vi "Read Tests.vi"() -> ()   [LabVIEW 2020]
uses:
  <vilib>/ActorFramework/Actor/Actor.lvclass
  FGV Map/Get Data/FGV Map Get Data (Variant).vi
  FGV Map/Get Data/FGV Map Get Data (String).vi
  FGV Map/Get Data/FGV Map Get Data (Bool).vi
  FGV Map/Get Data/FGV Map Get Data (DBL).vi
  FGV Map/Get Data/FGV Map Get Data (U32).vi
  FGV Map/Get Data/FGV Map Get Data (I32).vi
  FGV Map/Get Data/FGV Map Get Data (Path).vi
  FGV Map/Get Data/FGV Map Get Data (Class).vi
  FGV Map.lvlib
panel:
  out "Class2":bool
  out "Class1":bool
  out "Path":bool
  out "I32":bool
  out "U32":bool
  out "DBL":bool
  out "Bool":bool
  out "String":bool
  out "Variant":bool
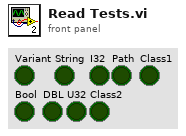
[diagram p1: front panel]
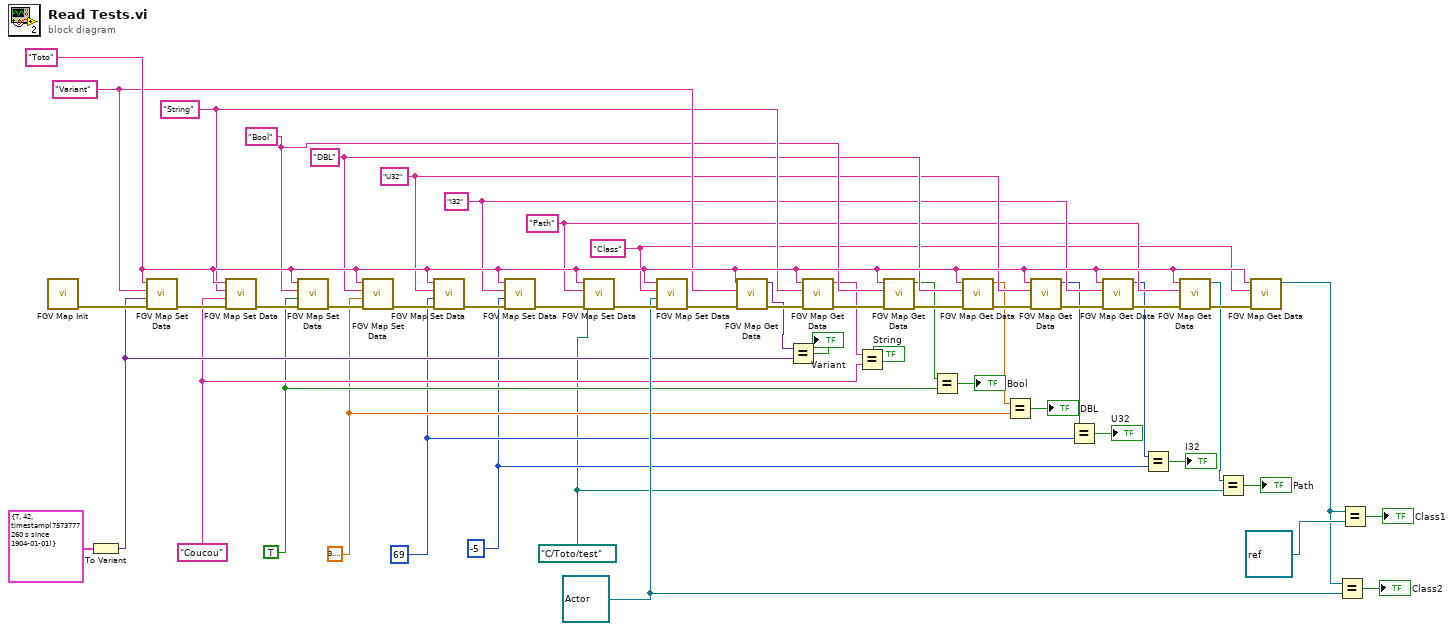
[diagram p0: block diagram]
diagram:
  w24 = refnum<class "Actor.lvclass"> refnum ("Actor")
  w27 = "Class" ("Data Key")
  w10 = path "C:/Toto/test"
  w14 = u32 69
  w12 = -5
  w16 = 3.141592653589793
  w18 = TRUE
  w20 = "Coucou"
  w28 = "Path" ("Data Key")
  w29 = "I32" ("Data Key")
  w30 = "U32" ("Data Key")
  w31 = "DBL" ("Instance Key")
  w32 = "Bool" ("Data Key")
  w33 = "String" ("Data Key")
  w34 = "Variant" ("Data Key")
  w35 = "Toto" ("Instance Key")
  n1 = call "FGV Map Init.vi"() -> ("error out"=w52:errorcluster)  [unwired: 11 in]
  n2 = To Variant(anything=cluster{bool, i32, timestamp} {TRUE, 42, timestamp(7573777260 s since 1904-01-01)}) -> (Variant=w22:variant)
  n3 = call "FGV Map Set Data.vi"("error in (no error)"=w52, "Data In"=w22, "Data Key"=w34, "Instance Key"=w35) -> ("error out"=w51:errorcluster)  [unwired: 5 in, 2 out]
  n4 = call "FGV Map Set Data.vi"("error in (no error)"=w51, "Data In"=w20, "Data Key"=w33, "Instance Key"=w35) -> ("error out"=w50:errorcluster)  [unwired: 5 in, 2 out]
  n5 = call "FGV Map Set Data.vi"("error in (no error)"=w50, "Data In"=w18, "Data Key"=w32, "Instance Key"=w35) -> ("error out"=w49:errorcluster)  [unwired: 5 in, 2 out]
  n6 = call "FGV Map Set Data.vi"("error in (no error)"=w49, "Data In"=w16, "Data Key"=w31, "Instance Key"=w35) -> ("error out"=w48:errorcluster)  [unwired: 5 in, 2 out]
  n7 = call "FGV Map Set Data.vi"("error in (no error)"=w48, "Data In"=w14, "Data Key"=w30, "Instance Key"=w35) -> ("error out"=w47:errorcluster)  [unwired: 5 in, 2 out]
  n8 = call "FGV Map Set Data.vi"("error in (no error)"=w47, "Data In"=w12, "Data Key"=w29, "Instance Key"=w35) -> ("error out"=w46:errorcluster)  [unwired: 5 in, 2 out]
  n9 = call "FGV Map Set Data.vi"("error in (no error)"=w46, "Data In"=w10, "Data Key"=w28, "Instance Key"=w35) -> ("error out"=w45:errorcluster)  [unwired: 5 in, 2 out]
  n10 = call "FGV Map Set Data.vi"("error in (no error)"=w45, "Data In"=w24, "Data Key"=w27, "Instance Key"=w35) -> ("error out"=w37:errorcluster)  [unwired: 5 in, 2 out]
  n11 = call-poly "FGV Map Get Data.vi"("error in (no error)"=w37, "Data Key"=w34, "Instance Key"=w35) -> ("error out"=w44:errorcluster, "Data Out"=w23:variant)  [unwired: 6 in, 1 out]
  n12 = Equal?(x=w23, y=w22) -> (x = y?=→"Variant":bool)
  n13 = call-poly "FGV Map Get Data.vi"("error in (no error)"=w44, "Data Key"=w33, "Instance Key"=w35) -> ("error out"=w43:errorcluster, "Data Out"=w21:string)  [unwired: 6 in, 1 out]
  n14 = Equal?(x=w21, y=w20) -> (x = y?=→"String":bool)
  n15 = call-poly "FGV Map Get Data.vi"("error in (no error)"=w43, "Data Key"=w32, "Instance Key"=w35) -> ("error out"=w42:errorcluster, "Data Out"=w19:bool)  [unwired: 6 in, 1 out]
  n16 = Equal?(x=w19, y=w18) -> (x = y?=→"Bool":bool)
  n17 = call-poly "FGV Map Get Data.vi"("error in (no error)"=w42, "Data Key"=w31, "Instance Key"=w35) -> ("error out"=w41:errorcluster, "Data Out"=w17:dbl)  [unwired: 6 in, 1 out]
  n18 = Equal?(x=w17, y=w16) -> (x = y?=→"DBL":bool)
  n19 = call-poly "FGV Map Get Data.vi"("error in (no error)"=w41, "Data Key"=w30, "Instance Key"=w35) -> ("error out"=w40:errorcluster, "Data Out"=w15:u32)  [unwired: 6 in, 1 out]
  n20 = Equal?(x=w15, y=w14) -> (x = y?=→"U32":bool)
  n21 = call-poly "FGV Map Get Data.vi"("error in (no error)"=w40, "Data Key"=w29, "Instance Key"=w35) -> ("error out"=w39:errorcluster, "Data Out"=w13:i32)  [unwired: 6 in, 1 out]
  n22 = Equal?(x=w13, y=w12) -> (x = y?=→"I32":bool)
  n23 = call-poly "FGV Map Get Data.vi"("error in (no error)"=w39, "Data Key"=w28, "Instance Key"=w35) -> ("error out"=w38:errorcluster, "Data Out"=w11:path)  [unwired: 6 in, 1 out]
  n24 = Equal?(x=w11, y=w10) -> (x = y?=→"Path":bool)
  n25 = call-poly "FGV Map Get Data.vi"("error in (no error)"=w38, "Data Key"=w27, "Instance Key"=w35) -> ("Data Out"=w25:refnum<class>)  [unwired: 6 in, 2 out]
  n26 = Equal?(x=w25, y=w24) -> (x = y?=→"Class2":bool)
  n27 = Equal?(x=w25, y=refnum<class> refnum ("LabVIEW Object")) -> (x = y?=→"Class1":bool)
